vi "Datei im Ordner des VI.vi"(11 "Dateiname":string="abc") -> (0 "EXE":bool, 2 "Ordner des Haupt-VIs":path, 3 "Dateipfad im Ordner des Haupt-VIs":path)   [LabVIEW 2015, in "Linearisierung v2.lvlib" / "Gasteiler.lvlib" / "HovaCal.lvlib"]
uses:
  HovaCal.lvlib
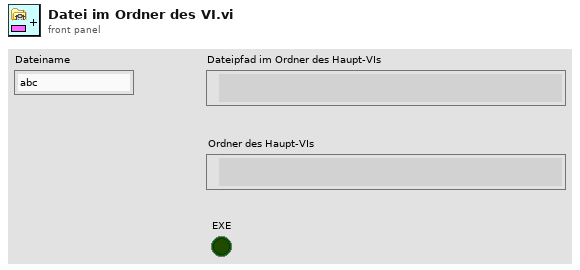
[diagram p1: front panel]
types:
  T1 = enum32{"invalid app kind", "Development System", "Run Time System", "Student Edition", "Embedded LabVIEW", "Evaluation", "Custom"}
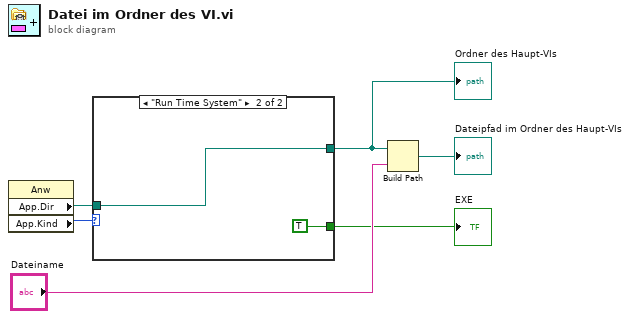
[diagram p0: block diagram]
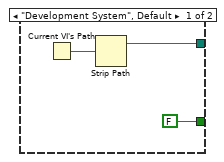
[diagram p2: hidden frame]
diagram:
  n1 = property class="Anw"() -> ("App.Dir"=w3:path, "App.Kind"=w4:T1)  [unwired: 2 in, 2 out]
  n2 = case shown="\"Run Time System\"" w4 {
    tunnel: w3 -> [_ w11]
    tunnel: [w9 w11] -> w2
    tunnel: [FALSE TRUE] -> w1
    frame "Development System", Default {
      n3 = Current VI's Path() -> (path=w7:path)
      n4 = Strip Path(path=w7) -> (stripped path=w9:path)  [unwired: 1 out]
    }
    frame "Run Time System" {
    }
  }
  "Ordner des Haupt-VIs" <- w2
  "EXE" <- w1
  n5 = Build Path(base path=w2, name or relative path="Dateiname") -> (appended path=→"Dateipfad im Ordner des Haupt-VIs":path)
